vi "MIPI_RFEE_Write Utility.vi"() -> ()   [LabVIEW 2013]
doc: "This VI demonstaits how to write to and read back data from a MIPI device. To run this VI:\n1) Change Resource name to the name of your HSDIO card\n2) The MIPI clock will run at <Sample Clock Rate>/<Oversample Factor>. This is 26 MHz (full rate). If your device should be run at a slower rate, decrease the sample clock rate and (or) increase the oversample rate.\n3. At 104MHz, the RTD value should be ~5 for a 1.5 meter cable. If you are running at a different clock rate or using a different length cable, adjust the RTD Compensation value so the MIPI data is stable at the falling edge of the clock. If you need futher timing adjustment, consider setting the data position to \"Delay from Sample Clock Rising Edge\" and configuring this delay."
uses:
  MIPI_RFFE/Ctrls/Configuration.ctl
  MIPI_RFFE/Ctrls/ClockDataChannels.ctl
  MIPI_RFFE/Ctrls/RegReadWrite.ctl
  <instrlib>/niHSDIO/niHSDIO.llb/niHSDIO_ctl Voltage Logic Family Values (Ring).ctl
  <instrlib>/niHSDIO/niHSDIO.llb/niHSDIO_ctl Sample Clock Source Values (ComboBox).ctl
  <instrlib>/niHSDIO/niHSDIO.llb/niHSDIO_ctl Data Position Values (Ring).ctl
  MIPI_RFFE/Ctrls/ExtendedRegReadWrite.ctl
  <instrlib>/niHSDIO/niHSDIO.llb/niHSDIO Configure Data Voltage Logic Family.vi
  <instrlib>/niHSDIO/niHSDIO.llb/niHSDIO Configure Initial State (String).vi
  <instrlib>/niHSDIO/niHSDIO.llb/niHSDIO Configure Idle State (String).vi
  <instrlib>/niHSDIO/niHSDIO.llb/niHSDIO Write Named Waveform (WDT).vi
panel:
  in  "logic family":T1=81 items=["5.0V Logic"=5, "3.3V Logic"=6, "2.5V Logic"=7, "1.8V Logic"=8, "1.5V Logic"=80, "1.2V Logic"=81]
  in  "channel list (all:\"\")":string="4,6,2"
  in  "delay (0.000)":dbl format="%.3f"
  in  "Register Read/Write":T2={"Slave Address"=7, "Register"=28, "Data"=128, "SetID_Pin_State"=enum."0"} {"Register" format="%.0x"; "Slave Address" max=15 format="%.0x"}
  out "Digital Waveform Graph":digitalwaveform(graph)={"t0"=timestamp(3585852840.1106524 s since 1904-01-01), "dt"=5e-07, "Y"={"transitions"=[], "data"=[[1, 0, 1, 0], [1, 0, 1, 0], [1, 0, 1, 0], [1, 0, 1, 0], [1, 0, 1, 0], [1, 0, 1, 0], [1, 0, 1, 0], [1, 0, 1, 0], [0, 0, 0, 0], [0, 0, 0, 0], [0, 0, 0, 0], [0, 0, 0, 0], [0, 0, 0, 0], [0, 0, 0, 0], [0, 0, 0, 0], [0, 0, 0, 0], [0, 1, 0, 1], [0, 1, 0, 1], [0, 1, 0, 1], [0, 1, 0, 1], [0, 0, 0, 0], [0, 0, 0, 0], [0, 0, 0, 0], [0, 0, 0, 0], [1, 1, 1, 1], [1, 1, 1, 1], [1, 1, 1, 1], [1, 1, 1, 1], [1, 0, 1, 0], [1, 0, 1, 0], [1, 0, 1, 0], [1, 0, 1, 0], [1, 1, 1, 1], [1, 1, 1, 1], [1, 1, 1, 1], [1, 1, 1, 1], [1, 0, 1, 0], [1, 0, 1, 0], [1, 0, 1, 0], [1, 0, 1, 0], [0, 1, 0, 1], [0, 1, 0, 1], [0, 1, 0, 1], [0, 1, 0, 1], [0, 0, 0, 0], [0, 0, 0, 0], [0, 0, 0, 0], [0, 0, 0, 0], [0, 1, 0, 1], [0, 1, 0, 1], [0, 1, 0, 1], [0, 1, 0, 1], [0, 0, 0, 0], [0, 0, 0, 0], [0, 0, 0, 0], [0, 0, 0, 0], [1, 1, 1, 1], [1, 1, 1, 1], [1, 1, 1, 1], [1, 1, 1, 1], [1, 0, 1, 0], [1, 0, 1, 0], [1, 0, 1, 0], [1, 0, 1, 0], [0, 1, 0, 1], [0, 1, 0, 1], [0, 1, 0, 1], [0, 1, 0, 1], [0, 0, 0, 0], [0, 0, 0, 0], [0, 0, 0, 0], [0, 0, 0, 0], [1, 1, 1, 1], [1, 1, 1, 1], [1, 1, 1, 1], [1, 1, 1, 1], [1, 0, 1, 0], [1, 0, 1, 0], [1, 0, 1, 0], [1, 0, 1, 0], [1, 1, 1, 1], [1, 1, 1, 1], [1, 1, 1, 1], [1, 1, 1, 1], [1, 0, 1, 0], [1, 0, 1, 0], [1, 0, 1, 0], [1, 0, 1, 0], [1, 1, 1, 1], [1, 1, 1, 1], [1, 1, 1, 1], [1, 1, 1, 1], [1, 0, 1, 0], [1, 0, 1, 0], [1, 0, 1, 0], [1, 0, 1, 0], [0, 1, 0, 1], [0, 1, 0, 1], [0, 1, 0, 1], [0, 1, 0, 1], [0, 0, 0, 0], [0, 0, 0, 0], [0, 0, 0, 0], [0, 0, 0, 0], [0, 1, 0, 1], [0, 1, 0, 1], [0, 1, 0, 1], [0, 1, 0, 1], [0, 0, 0, 0], [0, 0, 0, 0], [0, 0, 0, 0], [0, 0, 0, 0], [1, 1, 1, 1], [1, 1, 1, 1], [1, 1, 1, 1], [1, 1, 1, 1], [1, 0, 1, 0], [1, 0, 1, 0], [1, 0, 1, 0], [1, 0, 1, 0], [1, 1, 1, 1], [1, 1, 1, 1], [1, 1, 1, 1], [1, 1, 1, 1], [1, 0, 1, 0], [1, 0, 1, 0], [1, 0, 1, 0], [1, 0, 1, 0], [0, 1, 0, 1], [0, 1, 0, 1], [0, 1, 0, 1], [0, 1, 0, 1], [0, 0, 0, 0], [0, 0, 0, 0], [0, 0, 0, 0], [0, 0, 0, 0], [0, 1, 0, 1], [0, 1, 0, 1], [0, 1, 0, 1], [0, 1, 0, 1], [0, 0, 0, 0], [0, 0, 0, 0], [0, 0, 0, 0], [0, 0, 0, 0], [0, 1, 0, 1], [0, 1, 0, 1], [0, 1, 0, 1], [0, 1, 0, 1], [0, 0, 0, 0], [0, 0, 0, 0], [0, 0, 0, 0], [0, 0, 0, 0], [0, 1, 0, 1], [0, 1, 0, 1], [0, 1, 0, 1], [0, 1, 0, 1], [0, 0, 0, 0], [0, 0, 0, 0], [0, 0, 0, 0], [0, 0, 0, 0], [0, 1, 0, 1], [0, 1, 0, 1], [0, 1, 0, 1], [0, 1, 0, 1], [0, 0, 0, 0], [0, 0, 0, 0], [0, 0, 0, 0], [0, 0, 0, 0], [0, 1, 0, 1], [0, 1, 0, 1], [0, 1, 0, 1], [0, 1, 0, 1], [0, 0, 0, 0], [0, 0, 0, 0], [0, 0, 0, 0], [0, 0, 0, 0], [0, 1, 0, 1], [0, 1, 0, 1], [0, 1, 0, 1], [0, 1, 0, 1], [0, 0, 0, 0], [0, 0, 0, 0], [0, 0, 0, 0], [0, 0, 0, 0], [0, 1, 0, 1], [0, 1, 0, 1], [0, 1, 0, 1], [0, 1, 0, 1], [0, 0, 0, 0], [0, 0, 0, 0], [0, 0, 0, 0], [0, 0, 0, 0], [0, 1, 0, 1], [0, 1, 0, 1], [0, 1, 0, 1], [0, 1, 0, 1], [0, 0, 0, 0], [0, 0, 0, 0], [0, 0, 0, 0], [0, 0, 0, 0], [1, 0, 1, 0], [1, 0, 1, 0], [1, 0, 1, 0], [1, 0, 1, 0], [1, 0, 1, 0], [1, 0, 1, 0], [1, 0, 1, 0], [1, 0, 1, 0], [0, 0, 0, 0], [0, 0, 0, 0], [0, 0, 0, 0], [0, 0, 0, 0], [0, 0, 0, 0], [0, 0, 0, 0], [0, 0, 0, 0], [0, 0, 0, 0], [0, 1, 0, 1], [0, 1, 0, 1], [0, 1, 0, 1], [0, 1, 0, 1], [0, 0, 0, 0], [0, 0, 0, 0], [0, 0, 0, 0], [0, 0, 0, 0], [1, 1, 1, 1], [1, 1, 1, 1], [1, 1, 1, 1], [1, 1, 1, 1], [1, 0, 1, 0], [1, 0, 1, 0], [1, 0, 1, 0], [1, 0, 1, 0], [1, 1, 1, 1], [1, 1, 1, 1], [1, 1, 1, 1], [1, 1, 1, 1], [1, 0, 1, 0], [1, 0, 1, 0], [1, 0, 1, 0], [1, 0, 1, 0], [0, 1, 0, 1], [0, 1, 0, 1], [0, 1, 0, 1], [0, 1, 0, 1], [0, 0, 0, 0], [0, 0, 0, 0], [0, 0, 0, 0], [0, 0, 0, 0], [0, 1, 0, 1], [0, 1, 0, 1], [0, 1, 0, 1], [0, 1, 0, 1], [0, 0, 0, 0], [0, 0, 0, 0], [0, 0, 0, 0], [0, 0, 0, 0], [1, 1, 1, 1], [1, 1, 1, 1], [1, 1, 1, 1], [1, 1, 1, 1], [1, 0, 1, 0], [1, 0, 1, 0], [1, 0, 1, 0], [1, 0, 1, 0], [1, 1, 1, 1], [1, 1, 1, 1], [1, 1, 1, 1], [1, 1, 1, 1], [1, 0, 1, 0], [1, 0, 1, 0], [1, 0, 1, 0], [1, 0, 1, 0], [1, 1, 1, 1], [1, 1, 1, 1], [1, 1, 1, 1], [1, 1, 1, 1], [1, 0, 1, 0], [1, 0, 1, 0], [1, 0, 1, 0], [1, 0, 1, 0], [1, 1, 1, 1], [1, 1, 1, 1], [1, 1, 1, 1], [1, 1, 1, 1], [1, 0, 1, 0], [1, 0, 1, 0], [1, 0, 1, 0], [1, 0, 1, 0], [1, 1, 1, 1], [1, 1, 1, 1], [1, 1, 1, 1], [1, 1, 1, 1], [1, 0, 1, 0], [1, 0, 1, 0], [1, 0, 1, 0], [1, 0, 1, 0], [0, 1, 0, 1], [0, 1, 0, 1], [0, 1, 0, 1], [0, 1, 0, 1], [0, 0, 0, 0], [0, 0, 0, 0], [0, 0, 0, 0], [0, 0, 0, 0], [0, 1, 0, 1], [0, 1, 0, 1], [0, 1, 0, 1], [0, 1, 0, 1], [0, 0, 0, 0], [0, 0, 0, 0], [0, 0, 0, 0], [0, 0, 0, 0], [0, 1, 0, 1], [0, 1, 0, 1], [0, 1, 0, 1], [0, 1, 0, 1], [0, 0, 0, 0], [0, 0, 0, 0], [0, 0, 0, 0], [0, 0, 0, 0], [0, 1, 0, 1], [0, 1, 0, 1], [0, 1, 0, 1], [0, 1, 0, 1], [0, 0, 0, 0], [0, 0, 0, 0], [0, 0, 0, 0], [0, 0, 0, 0], [1, 1, 5, 1], [1, 1, 5, 1], [1, 1, 5, 1], [1, 1, 5, 1], [1, 0, 4, 0], [1, 0, 5, 0], [1, 0, 5, 0], [1, 0, 5, 0], [0, 1, 5, 1], [0, 1, 5, 1], [0, 1, 5, 1], [0, 1, 5, 1], [0, 0, 3, 0], [0, 0, 5, 0], [0, 0, 5, 0], [0, 0, 5, 0], [0, 1, 5, 1], [0, 1, 5, 1], [0, 1, 5, 1], [0, 1, 5, 1], [0, 0, 3, 0], [0, 0, 5, 0], [0, 0, 5, 0], [0, 0, 5, 0], [0, 1, 5, 1], [0, 1, 5, 1], [0, 1, 5, 1], [0, 1, 5, 1], [0, 0, 3, 0], [0, 0, 5, 0], [0, 0, 5, 0], [0, 0, 5, 0], [0, 1, 5, 1], [0, 1, 5, 1], [0, 1, 5, 1], [0, 1, 5, 1], [0, 0, 3, 0], [0, 0, 5, 0], [0, 0, 5, 0], [0, 0, 5, 0], [0, 1, 5, 1], [0, 1, 5, 1], [0, 1, 5, 1], [0, 1, 5, 1], [0, 0, 3, 0], [0, 0, 5, 0], [0, 0, 5, 0], [0, 0, 5, 0], [0, 1, 5, 1], [0, 1, 5, 1], [0, 1, 5, 1], [0, 1, 5, 1], [0, 0, 3, 0], [0, 0, 5, 0], [0, 0, 5, 0], [0, 0, 5, 0], [0, 1, 5, 1], [0, 1, 5, 1], [0, 1, 5, 1], [0, 1, 5, 1], [0, 0, 3, 0], [0, 0, 5, 0], [0, 0, 5, 0], [0, 0, 5, 0], [0, 1, 5, 1], [0, 1, 5, 1], [0, 1, 5, 1], [0, 1, 5, 1], [0, 0, 3, 0], [0, 0, 5, 0], [0, 0, 5, 0], [0, 0, 5, 0], [0, 1, 0, 1], [0, 1, 0, 1], [0, 1, 0, 1], [0, 1, 0, 1], [0, 0, 0, 0], [0, 0, 0, 0], [0, 0, 0, 0], [0, 0, 0, 0]]}}
  in  "Configuratation":T3={"Samples to Allocate"=10000, "Oversample Factor"=1, "Clock Channel"=enum."0", "Data Channel"=enum."1"} {"Oversample Factor" min=1 max=254; "Samples to Allocate" min=1}
  in  "Sample Clock Rate":dbl=2000000.0 format="%#_6p"
  in  "Resource name":refnum<k15>="6556_0"
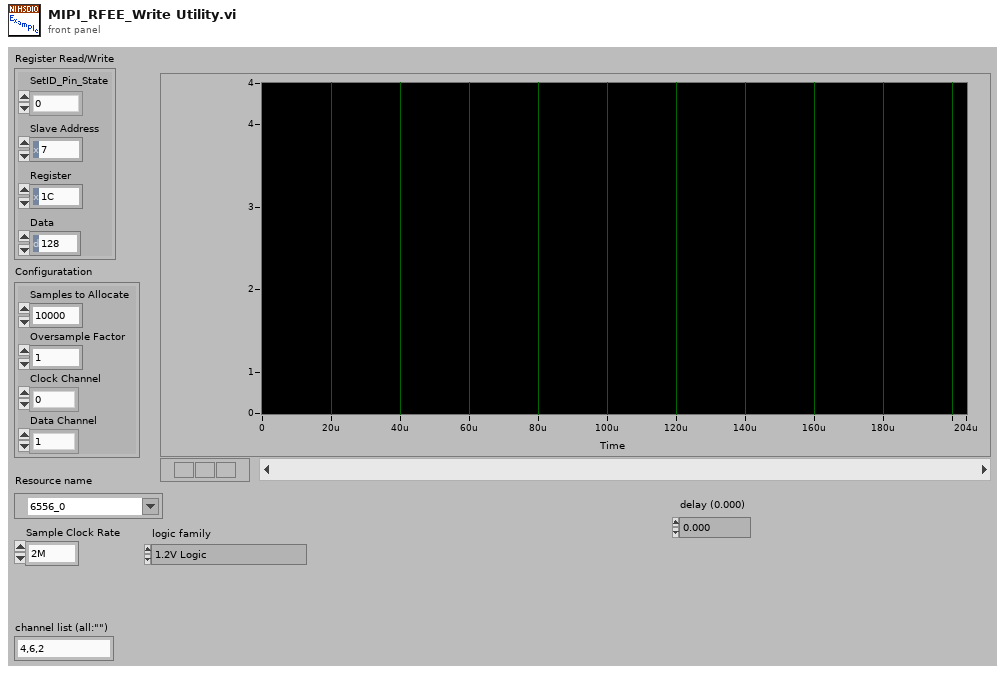
[diagram p1: front panel]
types:
  T1 = typedef "niHSDIO_ctl Voltage Logic Family Values (Ring).ctl" = i32
  T2 = typedef "RegReadWrite.ctl" = cluster{"Slave Address":u8, "Register":u8, "Data":u8, "SetID_Pin_State":enum16{"0", "1", "Z"}}
  T3 = typedef "Configuration.ctl" = cluster{"Samples to Allocate":i32, "Oversample Factor":u8, "Clock Channel":T4, "Data Channel":T4}
  T4 = typedef "ClockDataChannels.ctl" = enum16{"0", "1"}
  T5 = typedef "niHSDIO_ctl Data Position Values (Ring).ctl" = i32
  T6 = typedef "niHSDIO_ctl Sample Clock Source Values (ComboBox).ctl" = string
  T7 = typedef "RFFE_Data.ctl" = cluster{"Clock Channel":T4, "Data Channel":T4, "Oversample Factor":u8, "Zero Array":u8[], "One Array":u8[], "Z Array ":u8[], "H Array":u8[], "L Array":u8[], "X Array":u8[], "Toggle (high to low)":u8[]}
  T8 = typedef "ExtendedRegReadWrite.ctl" = cluster{"Slave Address":u8, "Register":u8, "Data":u8[]}
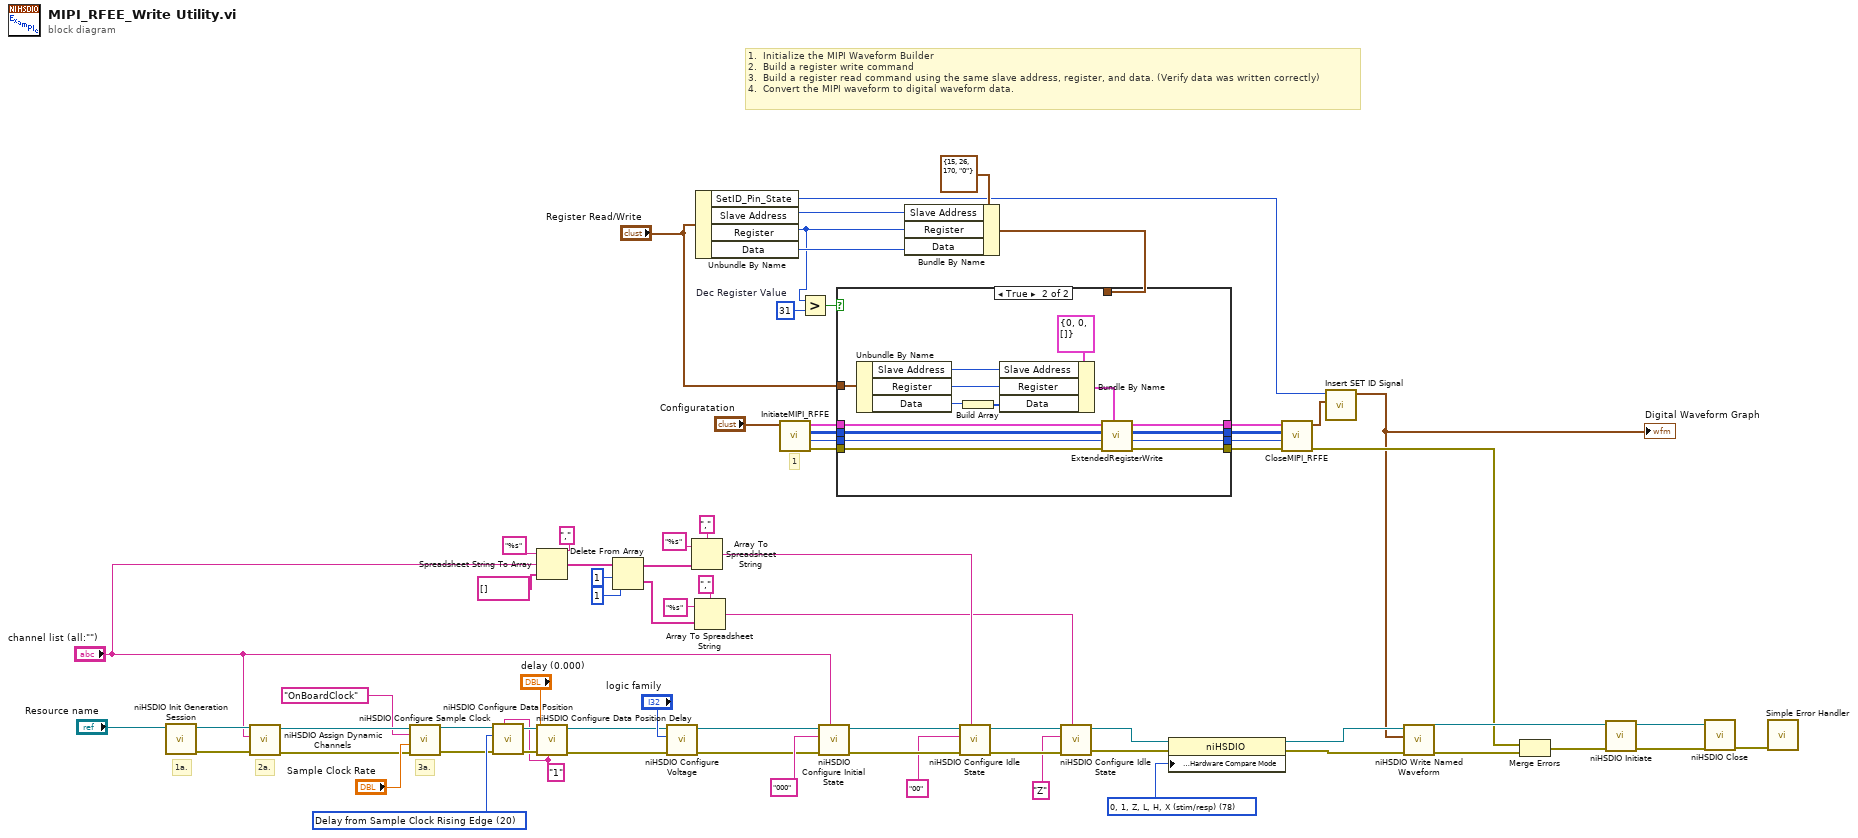
[diagram p0: block diagram]
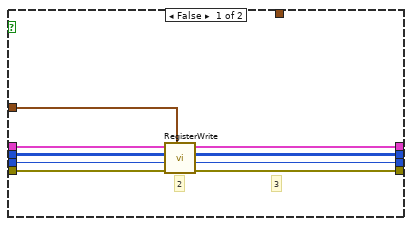
[diagram p2: hidden frame]
diagram:
  w35 = u8 31  # Dec Register Value
  w41 = T5 20 items=["Sample Clock Rising Edge"=18, "Sample Clock Falling Edge"=19, "Delay from Sample Clock Rising Edge"=20] ("position (rising edge)")
  w40 = "1" ("channel list (all:\"\")")
  w70 = 78 items=["0, 1 (binary)"=77, "0, 1, Z (tristate)"=83, "0, 1, Z, L, H, X (stim/resp)"=78, "L, H, X (resp only)"=79] ("Advanced:Supported Data States")
  # "1"
  # "1.  Initialize the MIPI Waveform Builder\n2.  Build a register write command\n3.  Build a register read command using the same slave address, register, and data. (Verify data was written correctly)\n4.  Convert the MIPI waveform to digital waveform data."
  # "3a."
  # "2a."
  # "1a."
  n1 = call <instrlib>:"niHSDIO Init Generation Session.vi"("resource name"="Resource name") -> ("error out"=w56:errorcluster, "instrument handle out"=w57:refnum<k15>)  [unwired: 9 in]
  n2 = call <instrlib>:"niHSDIO Assign Dynamic Channels.vi"("error in (no error)"=w56, "channel list (all:\"\")"="channel list (all:\"\")", "instrument handle"=w57) -> ("error out"=w68:errorcluster, "instrument handle out"=w69:refnum<k15>)  [unwired: 7 in]
  n3 = call <instrlib>:"niHSDIO Configure Sample Clock.vi"("error in (no error)"=w68, "clock rate (50MHz)"="Sample Clock Rate", "clock source (on board clock)"=T6 "OnBoardClock", "instrument handle"=w69) -> ("error out"=w23:errorcluster, "instrument handle out"=w22:refnum<k15>)  [unwired: 6 in]
  n4 = call <instrlib>:"niHSDIO Configure Data Position.vi"("channel list (all:\"\")"=w40, "error in (no error)"=w23, "position (rising edge)"=w41, "instrument handle"=w22) -> ("error out"=w43:errorcluster, "instrument handle out"=w42:refnum<k15>)  [unwired: 6 in]
  n5 = Spreadsheet String To Array(delimiter (Tab)=",", format string="%s", spreadsheet string="channel list (all:\"\")", array type (2D Dbl)=string[] []) -> (array=w19:string[])
  n6 = call <instrlib>:"niHSDIO Configure Data Position Delay.vi"("channel list (all:\"\")"=w40, "error in (no error)"=w43, "delay (0.000)"="delay (0.000)", "instrument handle"=w42) -> ("error out"=w46:errorcluster, "instrument handle out"=w45:refnum<k15>)  [unwired: 6 in]
  n7 = Delete From Array(array=w19, length=1, index=1) -> (deleted portion=w15:string[], array with subset deleted=w16:string[])
  n8 = call-poly <instrlib>:"niHSDIO Configure Voltage.vi"("error in (no error)"=w46, "logic family (3.3V logic)"="logic family", "instrument handle"=w45) -> ("error out"=w47:errorcluster, "instrument handle out"=w48:refnum<k15>)  [unwired: 7 in]
  n9 = Array To Spreadsheet String(delimiter (Tab)=",", array=w16, 3:"%s" ("format string")) -> (spreadsheet string=w9:string)
  n10 = Array To Spreadsheet String(delimiter (Tab)=",", array=w15, 3:"%s" ("format string")) -> (spreadsheet string=w3:string)
  n11 = Unbundle By Name("Register Read/Write") -> ("SetID_Pin_State"=w26:enum16{"0", "1", "Z"}, "Slave Address"=w38:u8, "Register"=w27:u8, "Data"=w34:u8)
  n12 = call "InitiateMIPI_RFFE.vi"("Configuratation In"="Configuratation") -> ("error out"=w62:errorcluster, "Number of Samples Out"=w61:i32, "Data Array"=w60:u8[][], "RFFE_Data"=w59:T7)  [unwired: 7 in]
  n13 = Greater?(x=w27, y=w35) -> (0:w33:bool)
  n14 = call-poly <instrlib>:"niHSDIO Configure Initial State.vi"("channel list"="channel list (all:\"\")", "error in (no error)"=w47, "initial state"="000" ("idle state"), "instrument handle"=w48) -> ("error out"=w50:errorcluster, "instrument handle out"=w49:refnum<k15>)  [unwired: 6 in]
  n15 = Bundle By Name(cluster=T2 {"Slave Address"=15, "Register"=26, "Data"=170, "SetID_Pin_State"=enum."0"} ("Register Read/Write"), "Slave Address"=w38, "Register"=w27, "Data"=w34) -> (w37:T2)
  n16 = case shown="True" w33 {
    tunnel: w62 -> [w82 w97]
    tunnel: w61 -> [w81 w94]
    tunnel: w60 -> [w80 w95]
    tunnel: w59 -> [w79 w96]
    tunnel: [w77 w86] -> w54
    tunnel: [w76 w85] -> w53
    tunnel: [w75 w84] -> w52
    tunnel: [w74 w83] -> w31
    tunnel: w37 -> [_ _]
    tunnel: "Register Read/Write" -> [w78 w92]
    frame False {
      # "3"
      # "2"
      n17 = call "RegisterWrite.vi"("Write Data"=w78, "error in (no error)"=w82, "Number of Samples In"=w81, "Data Array"=w80, "RFFE_Data"=w79) -> ("error out"=w74:errorcluster, "Number of Samples Out"=w75:i32, "Data Array Out"=w76:u8[][], "Configuratation Out"=w77:T7)  [unwired: 3 in]
    }
    frame True {
      n18 = Unbundle By Name(w92) -> ("Slave Address"=w91:u8, "Register"=w90:u8, "Data"=w89:u8)
      n19 = Build Array(w89) -> (w88:u8[])
      n20 = Bundle By Name(cluster=T8 {"Slave Address"=0, "Register"=0, "Data"=[]} ("Extended Read/Write"), "Slave Address"=w91, "Register"=w90, "Data"=w88) -> (w87:T8)
      n21 = call "ExtendedRegisterWrite.vi"("Extended Read/Write"=w87, "error in (no error)"=w97, "Number of Samples In"=w94, "Data Array"=w95, "RFFE_Data In"=w96) -> ("error out"=w83:errorcluster, "Number of Samples Out"=w84:i32, "Data Array Out"=w85:u8[][], "RFFE_Data Out"=w86:T7)  [unwired: 3 in]
    }
  }
  n22 = call-poly <instrlib>:"niHSDIO Configure Idle State.vi"("channel list"=w9, "error in (no error)"=w50, "idle state"="00", "instrument handle"=w49) -> ("error out"=w8:errorcluster, "instrument handle out"=w5:refnum<k15>)  [unwired: 6 in]
  n23 = call-poly <instrlib>:"niHSDIO Configure Idle State.vi"("channel list"=w3, "error in (no error)"=w8, "idle state"="Z", "instrument handle"=w5) -> ("error out"=w7:errorcluster, "instrument handle out"=w6:refnum<k15>)  [unwired: 6 in]
  n24 = property on="Property Node" class="niHSDIO"(reference=w6, error in=w7, "Advanced:Hardware Compare:Hardware Compare Mode"=w70) -> (reference out=w67:refnum<k15>, error out=w66:errorcluster)
  n25 = call "CloseMIPI_RFFE.vi"("error in (no error)"=w31, "Number of Samples"=w52, "Data Array"=w53, "RFFE_Data"=w54) -> ("error out"=w32:errorcluster, "Digital Waveform"=w25:digitalwaveform)  [unwired: 6 in]
  n26 = call "Insert SET ID Signal.vi"("Digital Waveform Graph"=w25, "SetID_Pin_State"=w26) -> ("Digital Waveform Graph 2"=w24:digitalwaveform)  [unwired: 9 in]
  "Digital Waveform Graph" <- w24
  n27 = call-poly <instrlib>:"niHSDIO Write Named Waveform.vi"("error in (no error)"=w66, "data"=w24, "instrument handle"=w67) -> ("error out"=w65:errorcluster, "instrument handle out"=w71:refnum<k15>)  [unwired: 7 in]
  n28 = Merge Errors(w32, w65) -> (w29:errorcluster)
  n29 = call <instrlib>:"niHSDIO Initiate.vi"("error in (no error)"=w29, "instrument handle"=w71) -> ("error out"=w28:errorcluster, "instrument handle out"=w58:refnum<k15>)  [unwired: 8 in]
  n30 = call <instrlib>:"niHSDIO Close.vi"("error in (no error)"=w28, "instrument handle"=w58) -> ("error out"=w30:errorcluster)  [unwired: 9 in]
  n31 = call <vilib>:"Simple Error Handler.vi"("error in (no error)"=w30) -> ()  [unwired: 4 in, 5 out]
